vi "target_gas.vi"   [LabVIEW 2011]
uses:
  Input - Cluster gas.ctl
  Output - Cluster gas.ctl
  <vilib>/Platform/TimedLoop/XDataNode/timing_clust.ctl
  <vilib>/Platform/TimedLoop/XDataNode/nitl_modes.ctl
  <vilib>/Platform/TimedLoop/XDataNode/wakeup.ctl
  <vilib>/Platform/TimedLoop/XDataNode/XDataNode.xnode
  <vilib>/Platform/TimedLoop/XDataNode/XDNodeRunTimeDep.lvlib
panel:
  # "The Network Variable Engine and Variable Client Support must be installed on the RT target\nfor this application to function properly. If the Network Variable Engine is not supported on\nthe target (e.g.  FP-2000 with <32MB of RAM), open the project and move the variable library\nto My Computer in the project. Doing this will deploy the variables to localhost but\nwill still require that Variable Client Support be installed on the RT target."
types:
  T1 = cluster{"GA1 ch4 [%]":dbl, "GA1 co2 [%]":dbl, "GA1 h2 [%]":dbl, "empty":bool, "measuring point":u8}
  T2 = typedef "XDNodeRunTimeDep.lvlib/timing_clust.ctl" = cluster{"Expected End [f-1]":u64, "Actual End [f-1]":u64, "Finished Late? [f-1]":bool, "Expected End [i-1]":u64, "Actual End [i-1]":u64, "Finished Late? [i-1]":bool, "Expected Start [i]":u64, "Actual Start [i]":u64, "Expected Start [f]":u64, "Actual Start [f]":u64, "Source Name":string, "Structure Name":string, "Period":i64, "Deadline":i64, "Offset":i64, "Start":i64, "Priority":i32, "Timeout":i32, "Mode":T3, "Wakeup Reason":T4, "Error":errorcluster, "Source Type":string, "Secondary Source Type":string, "Global End Time":u64, "Global Start Time":u64, "Frame Duration":u64, "Iteration Duration":u64, "Assigned CPU":i32, "I/O Scan Engine Mode":u32}
  T3 = typedef "XDNodeRunTimeDep.lvlib/nitl_modes.ctl" = enum32{"No Change", "Process missed periods, maintain original phase", "Discard missed periods, maintain original phase", "Process missed periods, ignore original phase", "Discard missed periods, ignore original phase"}
  T4 = typedef "XDNodeRunTimeDep.lvlib/wakeup.ctl" = enum32{"Normal", "Aborted", "Asynchronous wakeup", "Timing source error", "Timed loop error", "Timeout"}
  T5 = typedef "Input - Cluster gas.ctl" = cluster{"GM P-1":bool, "GM P-2":bool, "measuring point":u32, "measuring mode":u8, "GM-V1,2":bool, "GM-V3,4":bool, "GM-V5":bool, "measuring volume":u32}
  T6 = typedef "Output - Cluster gas.ctl" = cluster{"B2G2 MR V1.1 AUF":bool, "B2G2 MR V1.1 ZU":bool, "B2G2 MR V1 AUF":bool, "B2G2 MR V1 ZU":bool, "B2G1 T2 V1 AUF":bool, "B2G1 T2 V1 ZU":bool, "B2G1 T2 V1.1 AUF":bool, "B2G1 T2 V1.1 ZU":bool, "B2G2 T2 V1 AUF":bool, "B2G2 T2 V1 ZU":bool, "B2G2 T2 V1.1 ZU":bool, "B2G2 T2 V1.1 AUF":bool, "B2G1 MR V1 AUF":bool, "B2G1 MR V1 ZU":bool, "B2G1 MR V1.1 AUF":bool, "B2G1 MR V1.1 ZU":bool, "B2G1 HR V1 AUF":bool, "B2G1 HR V1 ZU":bool, "B2G1 HR V1.1 AUF":bool, "B2G1 HR V1.1 ZU":bool, "Fab1 HR V1 AUF":bool, "Fab1 HR V1 ZU":bool, "Fab1 HR V1.1 AUF":bool, "Fab1 HR V1.1 ZU":bool, "Fab1 MR V1 AUF":bool, "Fab1 MR V1 ZU":bool, "Fab1 MR V1.1 AUF":bool, "Fab1 MR V1.1 ZU":bool, "Fab1 BL V1 AUF":bool, "Fab1 BL V1 ZU":bool, "Fab1 BL V1.1 AUF":bool, "Fab1 BL V1.1 ZU":bool, "Fab2 HR V1 AUF":bool, "Fab2 HR V1 ZU":bool, "Fab2 HR V1.1 AUF":bool, "Fab2 HR V1.1 ZU":bool, "Fab2 MR V1 AUF":bool, "Fab2 MR V1 ZU":bool, "Fab2 MR V1.1 AUF":bool, "Fab2 MR V1.1 ZU":bool, "GA1 ch4 [%]":dbl, "GA1 co2 [%]":dbl, "GA1 h2 [%]":dbl, "GM P1 RUN":bool, "GM V-1 AUF":bool, "GM V-1 ZU":bool, "GM V-2 AUF":bool, "GM V-2 ZU":bool, "GM V-3 AUF":bool, "GM V-3 ZU":bool, "GM V-4 AUF":bool, "GM V-4 ZU":bool, "GM P2 RUN":bool, "GM GZ-1 [imp]":u32, "GM DS-2 [bar]":dbl, "GM DS-1 [bar]":dbl, "GM TS-1 [°C]":dbl, "GM TS-2[°C]":dbl, "gas_values":cluster{"timestamp":timestamp, "GM DS-2 [bar]":dbl, "GA1 ch4 [%]":dbl, "GA1 co2 [%]":dbl, "GA1 h2 [%]":dbl, "GM DS-1 [bar]":dbl, "GM TS-1 [°C]":dbl, "GM TS-2 [°C]":dbl, "GM GZ-1 [l]":dbl, "empty":bool, "measuring point":u8}, "measuring mode":u8}
  T7 = cluster{"STOP":bool, "measuring point":u32, "measuring mode t-1":u8, "measuring mode t-2":u8, "measuring volume":u32, "gas_values":cluster{"GA1 ch4 [%]":dbl, "GA1 co2 [%]":dbl, "GA1 h2 [%]":dbl, "empty":bool, "measuring point":u8}}
  T8 = cluster{"timestamp":timestamp, "GM DS-2 [bar]":dbl, "GA1 ch4 [%]":dbl, "GA1 co2 [%]":dbl, "GA1 h2 [%]":dbl, "GM DS-1 [bar]":dbl, "GM TS-1 [°C]":dbl, "GM TS-2 [°C]":dbl, "GM GZ-1 [l]":dbl, "empty":bool, "measuring point":u8}
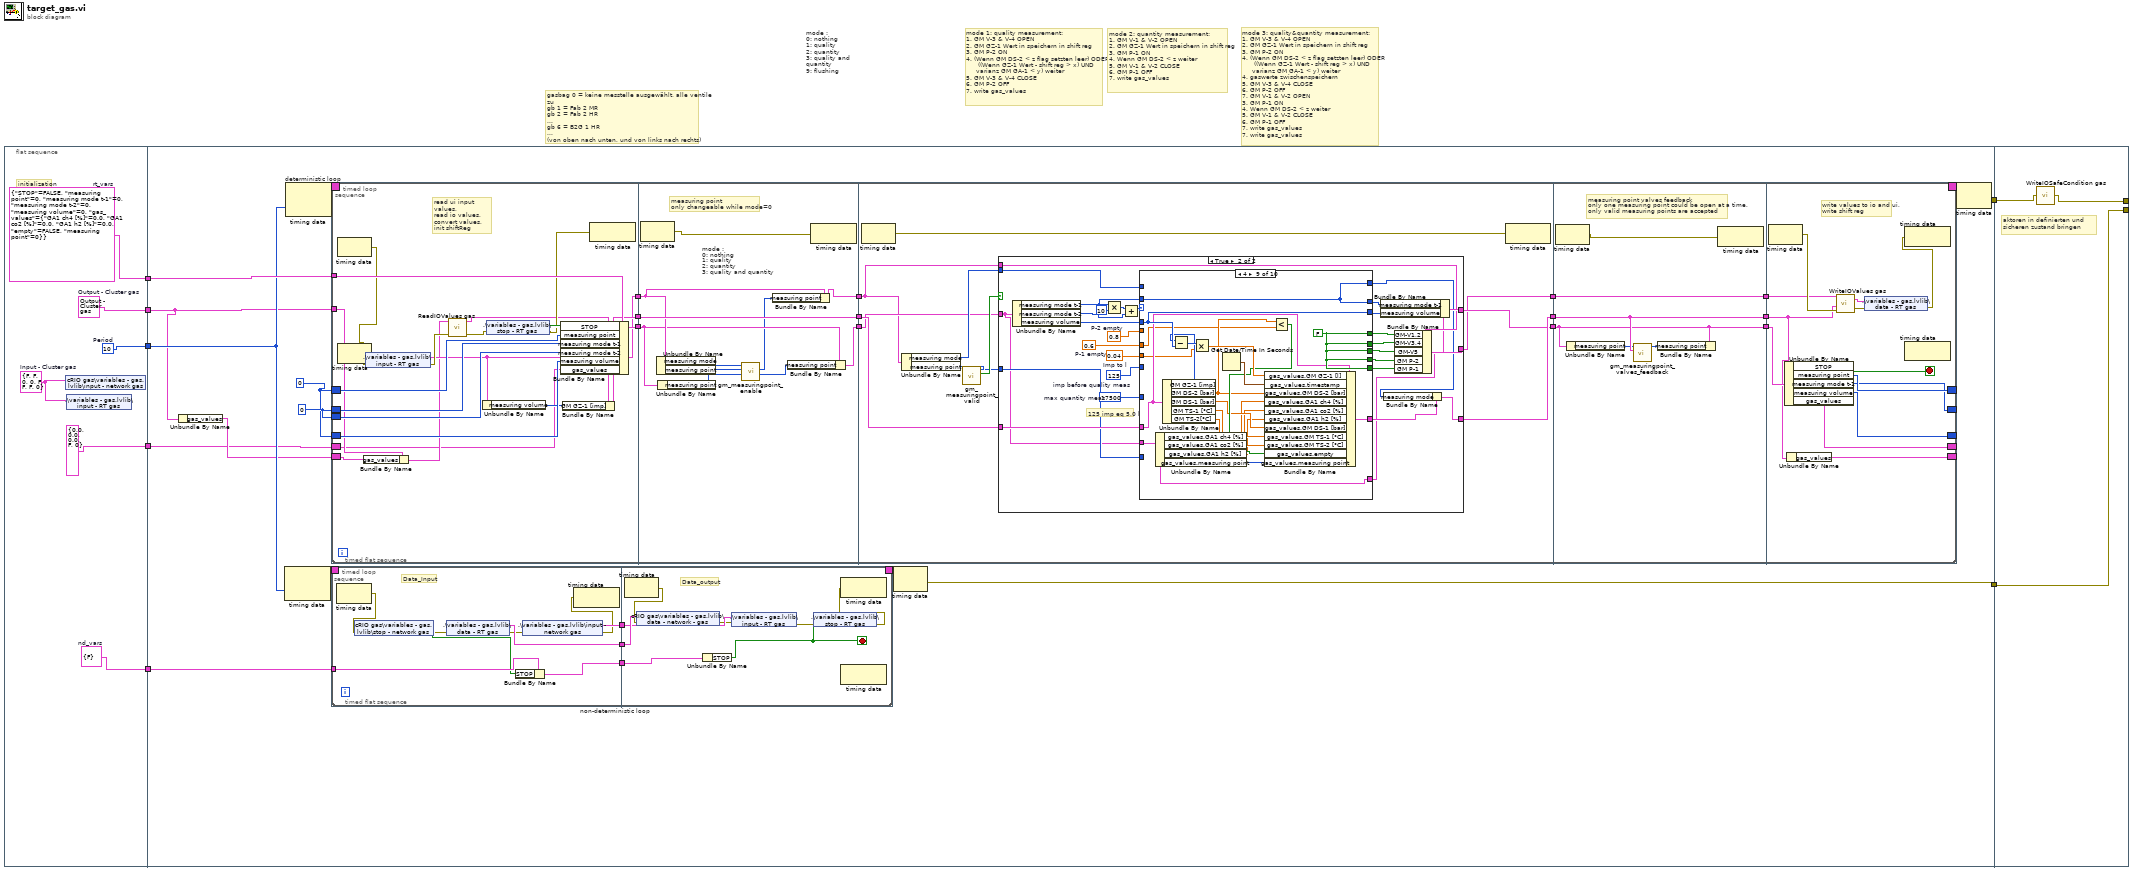
[diagram p0: block diagram]
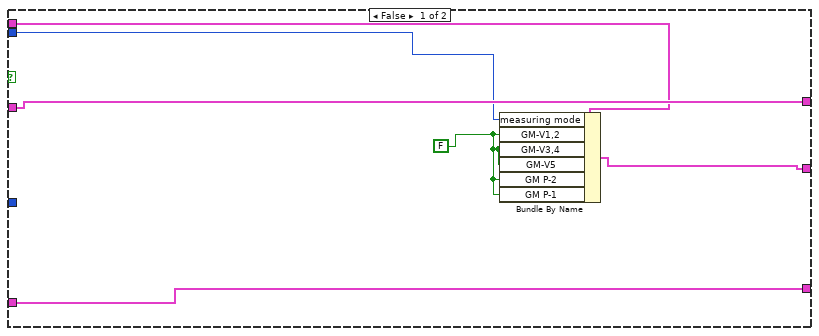
[diagram p2: hidden frame]
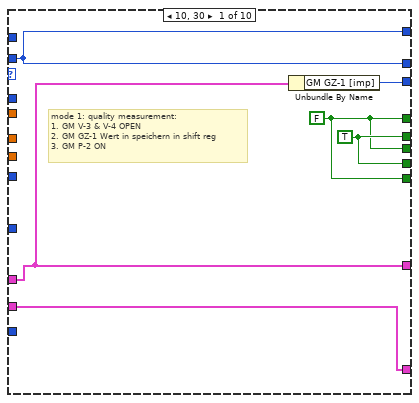
[diagram p3: hidden frame]
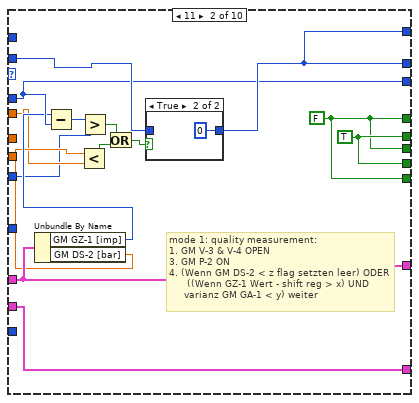
[diagram p4: hidden frame]
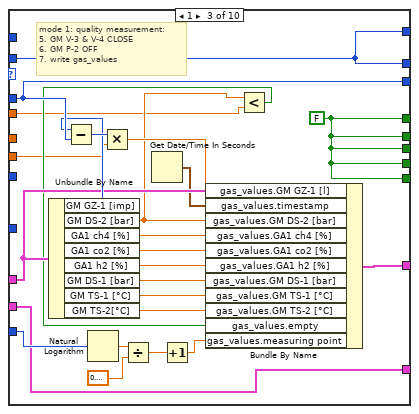
[diagram p6: hidden frame]
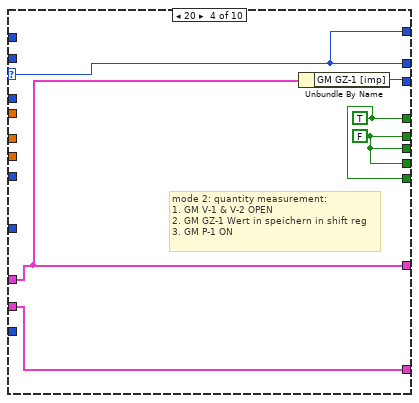
[diagram p7: hidden frame]
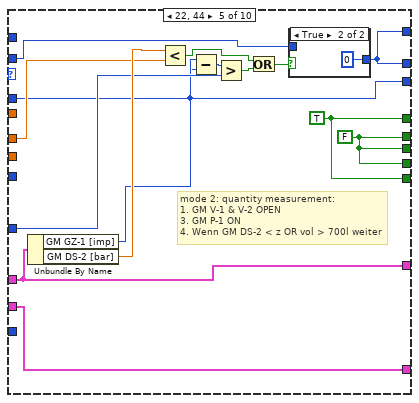
[diagram p8: hidden frame]
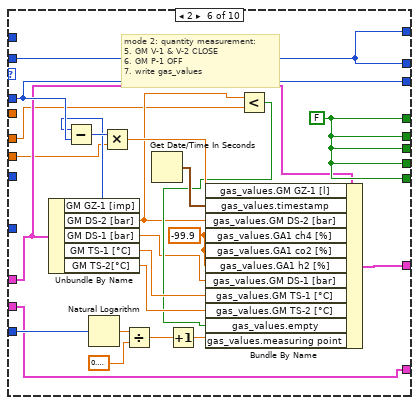
[diagram p10: hidden frame]
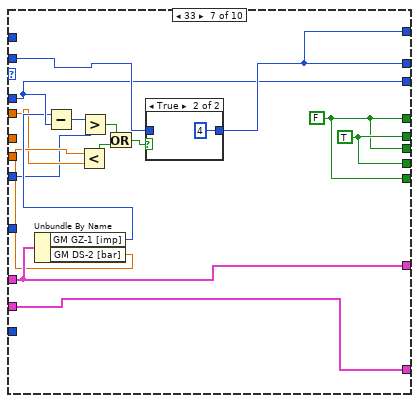
[diagram p11: hidden frame]
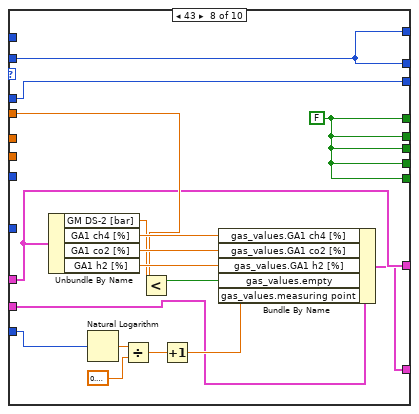
[diagram p13: hidden frame]
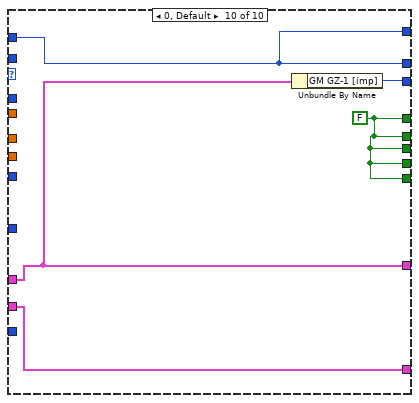
[diagram p14: hidden frame]
diagram:
  # "mode 3: quality&quantity measurement:\n1. GM V-3 & V-4 OPEN\n2. GM GZ-1 Wert in speichern in shift reg\n3. GM P-2 ON\n4. (Wenn GM DS-2 < z flag setzten leer) ODER\n      ((Wenn GZ-1 Wert - shift reg > x) UND\n     varianz GM GA-1 < y) weiter\n4. gaswerte zwischenspeichern\n5. GM V-3 & V-4 CLOSE\n6. GM P-2 OFF\n7. GM V-1 & V-2 OPEN\n3. GM P-1 ON\n4. Wenn GM DS-2 < z weiter\n5. GM V-1 & V-2 CLOSE\n6. GM P-1 OFF\n7. write gas_values\n7. write gas_values"
  # "mode 2: quantity measurement:\n1. GM V-1 & V-2 OPEN\n2. GM GZ-1 Wert in speichern in shift reg\n3. GM P-1 ON\n4. Wenn GM DS-2 < z weiter\n5. GM V-1 & V-2 CLOSE\n6. GM P-1 OFF\n7. write gas_values"
  # "mode :\n0: nothing\n1: quality\n2: quantity\n3: quality and quantity\n9: flushing"
  # "mode 1: quality measurement:\n1. GM V-3 & V-4 OPEN\n2. GM GZ-1 Wert in speichern in shift reg\n3. GM P-2 ON\n4. (Wenn GM DS-2 < z flag setzten leer) ODER\n      ((Wenn GZ-1 Wert - shift reg > x) UND\n     varianz GM GA-1 < y) weiter\n5. GM V-3 & V-4 CLOSE\n6. GM P-2 OFF\n7. write gas_values"
  # "gasbag 0 = keine messtelle ausgewählt, alle ventile zu\ngb 1 = Fab 2 MR\ngb 2 = Fab 2 HR \n...\ngb 6 = B2G 1 HR\n...\n(von oben nach unten, und von links nach rechts)"
  n1 = flat-sequence {
    tunnel: [w13] -> w7
    tunnel: [w12] -> w6
    tunnel: [w11] -> w5
    tunnel: [w9] -> w2
    tunnel: [T1 {"GA1 ch4 [%]"=0.0, "GA1 co2 [%]"=0.0, "GA1 h2 [%]"=0.0, "empty"=FALSE, "measuring point"=0} ("gas_values")] -> w1
    tunnel: w7 -> [w23]
    tunnel: w6 -> [w22]
    tunnel: w5 -> [w16]
    tunnel: [w21] -> w4
    tunnel: [w20] -> w3
    tunnel: w2 -> [w19]
    tunnel: w1 -> [w14]
    tunnel: w4 -> [w388]
    tunnel: w3 -> [w386]
    tunnel: [w387] -> _
    tunnel: [w388] -> _
    frame #0 {
      w9 = cluster{"STOP":bool} {"STOP"=FALSE}  # nd_vars
      w10 = T5 {"GM P-1"=FALSE, "GM P-2"=FALSE, "measuring point"=0, "measuring mode"=0, "GM-V1,2"=FALSE, "GM-V3,4"=FALSE, "GM-V5"=FALSE, "measuring volume"=0}  # Input - Cluster gas
      w11 = T6 {"B2G2 MR V1.1 AUF"=FALSE, "B2G2 MR V1.1 ZU"=FALSE, "B2G2 MR V1 AUF"=FALSE, "B2G2 MR V1 ZU"=FALSE, "B2G1 T2 V1 AUF"=FALSE, "B2G1 T2 V1 ZU"=FALSE, "B2G1 T2 V1.1 AUF"=FALSE, "B2G1 T2 V1.1 ZU"=FALSE, "B2G2 T2 V1 AUF"=FALSE, "B2G2 T2 V1 ZU"=FALSE, "B2G2 T2 V1.1 ZU"=FALSE, "B2G2 T2 V1.1 AUF"=FALSE, "B2G1 MR V1 AUF"=FALSE, "B2G1 MR V1 ZU"=FALSE, "B2G1 MR V1.1 AUF"=FALSE, "B2G1 MR V1.1 ZU"=FALSE, "B2G1 HR V1 AUF"=FALSE, "B2G1 HR V1 ZU"=FALSE, "B2G1 HR V1.1 AUF"=FALSE, "B2G1 HR V1.1 ZU"=FALSE, "Fab1 HR V1 AUF"=FALSE, "Fab1 HR V1 ZU"=FALSE, "Fab1 HR V1.1 AUF"=FALSE, "Fab1 HR V1.1 ZU"=FALSE, "Fab1 MR V1 AUF"=FALSE, "Fab1 MR V1 ZU"=FALSE, "Fab1 MR V1.1 AUF"=FALSE, "Fab1 MR V1.1 ZU"=FALSE, "Fab1 BL V1 AUF"=FALSE, "Fab1 BL V1 ZU"=FALSE, "Fab1 BL V1.1 AUF"=FALSE, "Fab1 BL V1.1 ZU"=FALSE, "Fab2 HR V1 AUF"=FALSE, "Fab2 HR V1 ZU"=FALSE, "Fab2 HR V1.1 AUF"=FALSE, "Fab2 HR V1.1 ZU"=FALSE, "Fab2 MR V1 AUF"=FALSE, "Fab2 MR V1 ZU"=FALSE, "Fab2 MR V1.1 AUF"=FALSE, "Fab2 MR V1.1 ZU"=FALSE, "GA1 ch4 [%]"=0.0, "GA1 co2 [%]"=0.0, "GA1 h2 [%]"=0.0, "GM P1 RUN"=FALSE, "GM V-1 AUF"=FALSE, "GM V-1 ZU"=FALSE, "GM V-2 AUF"=FALSE, "GM V-2 ZU"=FALSE, "GM V-3 AUF"=FALSE, "GM V-3 ZU"=FALSE, "GM V-4 AUF"=FALSE, "GM V-4 ZU"=FALSE, "GM P2 RUN"=FALSE, "GM GZ-1 [imp]"=0, "GM DS-2 [bar]"=0.0, "GM DS-1 [bar]"=0.0, "GM TS-1 [°C]"=0.0, "GM TS-2[°C]"=0.0, "gas_values"={"timestamp"=timestamp(0 s since 1904-01-01), "GM DS-2 [bar]"=0.0, "GA1 ch4 [%]"=0.0, "GA1 co2 [%]"=0.0, "GA1 h2 [%]"=0.0, "GM DS-1 [bar]"=0.0, "GM TS-1 [°C]"=0.0, "GM TS-2 [°C]"=0.0, "GM GZ-1 [l]"=0.0, "empty"=FALSE, "measuring point"=0}, "measuring mode"=0}  # Output - Cluster gas
      w13 = T7 {"STOP"=FALSE, "measuring point"=0, "measuring mode t-1"=0, "measuring mode t-2"=0, "measuring volume"=0, "gas_values"={"GA1 ch4 [%]"=0.0, "GA1 co2 [%]"=0.0, "GA1 h2 [%]"=0.0, "empty"=FALSE, "measuring point"=0}}  # rt_vars
      w12 = i64 10  # Period
      # "initialization"
      n2 = shared-variable "cRIO gas\\variables - gas.lvlib\\input - network gas"(w10) -> ()  [unwired: 1 in, 1 out]
      n3 = shared-variable ".\\variables - gas.lvlib\\input - RT gas"(w10) -> ()  [unwired: 1 in, 1 out]
    }
    frame #1 {
      w18 = u8 0 ("measuring point")
      w17 = u32 0 ("measuring point")
      n4 = Unbundle By Name(w16) -> ("gas_values"=w15:T8)
      n5 = node-c288 ("Input Node")(w22) -> (w25:T2)  [unwired: 1 in]
      n6 = node-c288 ("Input Node")(w22) -> (w27:T2)  [unwired: 1 in]
      n7 = timed-loop "non-deterministic loop" {
        timing: w25 -> [_]
        timing-out: [_] -> w24
        tunnel: w19 -> [w28]
        stop <- w51 stop-if-true
        n8 = timed-sequence {
          timing: _ -> [_]
          timing-out: _ -> [_]
          tunnel: w28 -> [w30]
          n9 = timed-flat-sequence {
            tunnel: [w38] -> w32
            tunnel: [w39] -> w31
            tunnel: w30 -> [w41]
            tunnel: [w40] -> w29
            tunnel: w31 -> [w52]
            tunnel: w32 -> [w53]
            tunnel: w29 -> [w54]
            frame #0 {
              # "Data_Input"
              n10 = node-c288() -> (w36:errorcluster)  [unwired: 1 in]
              n11 = shared-variable "cRIO gas\\variables - gas.lvlib\\stop - network gas"(error in=w36) -> (w37:bool, error out=w35:errorcluster)
              n12 = shared-variable ".\\variables - gas.lvlib\\data - RT gas"(error in=w35) -> (w38:T6, error out=w34:errorcluster)
              n13 = Bundle By Name(cluster=w41, "STOP"=w37) -> (w40:cluster{"STOP":bool})
              n14 = shared-variable ".\\variables - gas.lvlib\\input - network gas"(error in=w34) -> (w39:T5, error out=w33:errorcluster)
              n15 = node-c288(w33) -> ()  [unwired: 1 out]
            }
            frame #1 {
              # "Data_output"
              n16 = node-c288() -> (w50:errorcluster)  [unwired: 1 in]
              n17 = shared-variable "cRIO gas\\variables - gas.lvlib\\data - network - gas"(w53, error in=w50) -> (error out=w49:errorcluster)
              n18 = Unbundle By Name(w54) -> ("STOP"=w51:bool)
              n19 = shared-variable ".\\variables - gas.lvlib\\input - RT gas"(w52, error in=w49) -> (error out=w48:errorcluster)
              n20 = shared-variable ".\\variables - gas.lvlib\\stop - RT gas"(w51, error in=w48) -> (error out=w47:errorcluster)
              n21 = node-c288(w47) -> ()  [unwired: 1 out]
            }
          }
        }
        n22 = node-c288() -> ()  [unwired: 1 in, 1 out]
        n23 = node-c288() -> ()  [unwired: 1 in, 1 out]
      }
      n24 = timed-loop "deterministic loop" {
        timing: w27 -> [_]
        timing-out: [_] -> w26
        tunnel: w23 -> [w79]
        tunnel: w16 -> [w78]
        shift-right: [w77] -> _
        shift-left: w17 -> [w76]
        shift-right: [w75] -> _
        shift-left: w18 -> [w74]
        shift-left: w18 -> [w73]
        shift-right: [w72] -> _
        shift-left: w17 -> [w71]
        shift-right: [w70] -> _
        shift-left: w15 -> [w69]
        shift-right: [w68] -> _
        shift-left: w14 -> [w67]
        stop <- w370 stop-if-true
        n25 = timed-sequence {
          timing: _ -> [_]
          timing-out: _ -> [_]
          tunnel: w79 -> [w104]
          tunnel: w78 -> [w103]
          tunnel: [w96] -> w77
          tunnel: w76 -> [w95]
          tunnel: [w88] -> w75
          tunnel: w74 -> [w87]
          tunnel: w73 -> [w86]
          tunnel: [w85] -> w72
          tunnel: w71 -> [w84]
          tunnel: [w83] -> w70
          tunnel: w69 -> [w82]
          tunnel: [w81] -> w68
          tunnel: w67 -> [w80]
          n26 = timed-flat-sequence {
            tunnel: w104 -> [w123]
            tunnel: w103 -> [w108]
            tunnel: [w110] -> w102
            tunnel: [w119] -> w101
            tunnel: [w111] -> w100
            tunnel: w95 -> [w115]
            tunnel: w87 -> [w114]
            tunnel: w86 -> [w113]
            tunnel: w84 -> [w112]
            tunnel: w82 -> [w106]
            tunnel: w80 -> [w105]
            tunnel: w102 -> [w137]
            tunnel: [w130] -> w94
            tunnel: w101 -> [w134]
            tunnel: [w132] -> w92
            tunnel: w100 -> [w139]
            tunnel: [w139] -> w90
            tunnel: w94 -> [w147]
            tunnel: [w146] -> w93
            tunnel: w92 -> [w149]
            tunnel: [w148] -> w91
            tunnel: w90 -> [w151]
            tunnel: [w150] -> w89
            tunnel: w93 -> [w355]
            tunnel: [w355] -> w99
            tunnel: w91 -> [w350]
            tunnel: [w350] -> w98
            tunnel: w89 -> [w353]
            tunnel: [w353] -> w97
            tunnel: w99 -> [w367]
            tunnel: w98 -> [w371]
            tunnel: w97 -> [w363]
            tunnel: [w366] -> w96
            tunnel: [w365] -> w88
            tunnel: [w364] -> w85
            tunnel: [w362] -> w83
            tunnel: [w361] -> w81
            frame #0 {
              # "read ui input values,\nread io values,\nconvert values,\ninit shiftReg"
              n27 = node-c288 ("Output Node")() -> (w117:errorcluster)  [unwired: 1 in]
              n28 = Bundle By Name(cluster=w108, "gas_values"=w106) -> (w107:T6)
              n29 = shared-variable ".\\variables - gas.lvlib\\input - RT gas"(error in=w117) -> (w110:T5, error out=w116:errorcluster)
              n30 = call "ReadIOValues gas.vi"("error in"=w116, "Output - Cluster gas"=w107) -> ("error out"=w120:errorcluster, "Output - Cluster gas"=w118:T6)  [unwired: 2 in]
              n31 = Unbundle By Name(w110) -> ("measuring volume"=w109:u32)
              n32 = shared-variable ".\\variables - gas.lvlib\\stop - RT gas"(error in=w120) -> (w122:bool, error out=w121:errorcluster)
              n33 = Bundle By Name(cluster=w123, "STOP"=w122, "measuring point"=w115, "measuring mode t-1"=w114, "measuring mode t-2"=w113, "measuring volume"=w112, "gas_values"=w105) -> (w119:T7)
              n34 = Bundle By Name(cluster=w118, "GM GZ-1 [imp]"=w109) -> (w111:T6)
              n35 = node-c288 ("Input Node")(w121) -> ()  [unwired: 1 out]
            }
            frame #1 {
              # "mode :\n0: nothing\n1: quality\n2: quantity\n3: quality and quantity"
              # "measuring point\nonly changeable while mode=0"
              n36 = node-c288() -> (w138:errorcluster)  [unwired: 1 in]
              n37 = Unbundle By Name(w137) -> ("measuring mode"=w136:u8, "measuring point"=w135:u32)
              n38 = Unbundle By Name(w134) -> ("measuring point"=w133:u32)
              n39 = call "gm_measuringpoint_enable.vi"("shift reg"=w133, "measuring point"=w135, "measuring mode"=w136) -> ("shift reg out"=w131:u32, "measuring point"=w129:u32)  [unwired: 6 in]
              n40 = Bundle By Name(cluster=w137, "measuring point"=w129) -> (w130:T5)
              n41 = Bundle By Name(cluster=w134, "measuring point"=w131) -> (w132:T7)
              n42 = node-c288(w138) -> ()  [unwired: 1 out]
            }
            frame #2 {
              n43 = node-c288() -> (w155:errorcluster)  [unwired: 1 in]
              n44 = Unbundle By Name(w147) -> ("measuring mode"=w152:u8, "measuring point"=w153:u32)
              n45 = call "gm_measuringpoint_valid.vi"("measuring point in"=w153) -> ("Boolean"=w154:bool, "measuring point out"=w145:u32)  [unwired: 9 in]
              n46 = case shown="True" w154 {
                tunnel: w152 -> [w156 w190]
                tunnel: w151 -> [w161 w186]
                tunnel: [w161 w171] -> w150
                tunnel: w149 -> [w160 w163]
                tunnel: [w160 w182] -> w148
                tunnel: w147 -> [w159 w174]
                tunnel: [w158 w173] -> w146
                tunnel: w145 -> [_ w169]
                frame False {
                  w157 = FALSE ("GM-V3,4")
                  n47 = Bundle By Name(cluster=w159, "measuring mode"=w156, "GM-V1,2"=w157, "GM-V3,4"=w157, "GM-V5"=w157, "GM P-2"=w157, "GM P-1"=w157) -> (w158:T5)
                }
                frame True {
                  w164 = u32 17500  # max quantity meas
                  w165 = u32 125  # imp before quality meas
                  w166 = 0.6  # P-1 empty
                  w167 = 0.8  # P-2 empty
                  w168 = 0.04  # Imp to l
                  # "125 imp eq 5,0 l"
                  n48 = Unbundle By Name(w163) -> ("measuring mode t-1"=w185:u8, "measuring mode t-2"=w184:u8, "measuring volume"=w183:u32)
                  n49 = Multiply(x=w185, y=u8 10) -> (x*y=w189:u8)
                  n50 = Add(x=w189, y=w184) -> (x+y=w188:u8)
                  n51 = case shown="4" w188 {
                    selector: w188 -> [_ _ _ w244 _ _ _ _ _ _]
                    tunnel: w190 -> [_ _ _ _ _ _ _ _ _ w344]
                    tunnel: [w194 w208 w237 w244 w257 w283 w296 w317 w338 w344] -> w181
                    tunnel: [w195 w210 w238 w243 w259 w284 w298 w318 w339 w343] -> w179
                    tunnel: [w196 w211 w238 w242 w254 w284 w299 w318 w339 w343] -> w178
                    tunnel: [w195 w210 w238 w242 w254 w284 w298 w318 w339 w343] -> w177
                    tunnel: [w194 w208 w237 w244 w257 w283 w296 w317 w338 w344] -> w170
                    tunnel: [w192 w207 w236 w240 w247 w282 w295 w316 w337 w341] -> w180
                    tunnel: [w196 w211 w238 w242 w254 w284 w299 w318 w339 w343] -> w176
                    tunnel: [w195 w210 w238 w243 w259 w284 w298 w318 w339 w343] -> w175
                    tunnel: w183 -> [_ w207 w236 _ w247 w282 w295 w316 w337 _]
                    tunnel: w185 -> [w194 w209 w237 _ w258 w283 w297 w317 w338 _]
                    tunnel: w186 -> [w193 w202 w232 w241 w256 w278 w290 w304 w333 w342]
                    tunnel: [w193 w202 w233 w241 w256 w279 w290 w304 w334 w342] -> w172
                    tunnel: w169 -> [_ _ w221 _ _ w267 _ w309 _ _]
                    tunnel: w168 -> [_ _ w216 _ _ w263 _ _ w324 _]
                    tunnel: w167 -> [_ w199 w215 _ _ _ w287 w305 _ _]
                    tunnel: w166 -> [_ _ _ _ w253 w264 _ _ w325 _]
                    tunnel: w165 -> [_ w198 _ _ _ _ w286 _ _ _]
                    tunnel: w164 -> [_ _ _ _ w249 _ _ _ _ _]
                    tunnel: w163 -> [w191 w197 w214 w239 w245 w262 w285 w303 w323 w340]
                    tunnel: [w191 w197 w214 w239 w245 w262 w285 w302 w323 w340] -> w162
                    frame 10, 30 {
                      w195 = FALSE ("GM-V3,4")
                      w196 = TRUE ("GM-V3,4")
                      # "mode 1: quality measurement:\n1. GM V-3 & V-4 OPEN\n2. GM GZ-1 Wert in speichern in shift reg\n3. GM P-2 ON"
                      n52 = Unbundle By Name(w193) -> ("GM GZ-1 [imp]"=w192:u32)
                    }
                    frame 11 {
                      w210 = FALSE ("GM-V3,4")
                      w211 = TRUE ("GM-V3,4")
                      # "mode 1: quality measurement:\n1. GM V-3 & V-4 OPEN\n3. GM P-2 ON\n4. (Wenn GM DS-2 < z flag setzten leer) ODER\n      ((Wenn GZ-1 Wert - shift reg > x) UND\n     varianz GM GA-1 < y) weiter"
                      n53 = Unbundle By Name(w202) -> ("GM GZ-1 [imp]"=w201:u32, "GM DS-2 [bar]"=w200:dbl)
                      n54 = Subtract(x=w201, y=w207) -> (x-y=w206:u32)
                      n55 = Less?(x=w200, y=w199) -> (x < y?=w203:bool)
                      n56 = Greater?(x=w206, y=w198) -> (0:w204:bool)
                      n57 = Or(x=w204, y=w203) -> (x .or. y?=w205:bool)
                      n58 = case shown="True" w205 {
                        tunnel: w209 -> [w212 _]
                        tunnel: [w212 u8 0 ("measuring mode t-1")] -> w208
                        frame False {
                        }
                        frame True {
                        }
                      }
                    }
                    frame 1 {
                      w238 = FALSE ("GM-V3,4")
                      # "mode 1: quality measurement:\n5. GM V-3 & V-4 CLOSE\n6. GM P-2 OFF\n7. write gas_values"
                      n59 = Unbundle By Name(w232) -> ("GM GZ-1 [imp]"=w234:u32, "GM DS-2 [bar]"=w218:dbl, "GA1 ch4 [%]"=w229:dbl, "GA1 co2 [%]"=w228:dbl, "GA1 h2 [%]"=w227:dbl, "GM DS-1 [bar]"=w217:dbl, "GM TS-1 [°C]"=w226:dbl, "GM TS-2[°C]"=w225:dbl)
                      n60 = Subtract(x=w234, y=w236) -> (x-y=w235:u32)
                      n61 = Natural Logarithm(1:w221) -> (0:w223:dbl)
                      n62 = Multiply(x=w235, y=w216) -> (x*y=w230:dbl)
                      n63 = Divide(x=w223, y=0.6931471805599453) -> (x/y=w220:dbl)
                      n64 = Get Date/Time In Seconds ("timestamp")() -> (seconds since 1Jan1904=w231:timestamp)
                      n65 = Increment(x=w220) -> (x+1=w219:dbl)
                      n66 = Less?(x=w218, y=w215) -> (x < y?=w224:bool)
                      n67 = Bundle By Name(cluster=w232, "gas_values.GM GZ-1 [l]"=w230, "gas_values.timestamp"=w231, "gas_values.GM DS-2 [bar]"=w218, "gas_values.GA1 ch4 [%]"=w229, "gas_values.GA1 co2 [%]"=w228, "gas_values.GA1 h2 [%]"=w227, "gas_values.GM DS-1 [bar]"=w217, "gas_values.GM TS-1 [°C]"=w226, "gas_values.GM TS-2 [°C]"=w225, "gas_values.empty"=w224, "gas_values.measuring point"=w219) -> (w233:T6)
                    }
                    frame 20 {
                      w242 = FALSE ("GM-V3,4")
                      w243 = TRUE ("GM-V3,4")
                      # "mode 2: quantity measurement:\n1. GM V-1 & V-2 OPEN\n2. GM GZ-1 Wert in speichern in shift reg\n3. GM P-1 ON"
                      n68 = Unbundle By Name(w241) -> ("GM GZ-1 [imp]"=w240:u32)
                    }
                    frame 22, 44 {
                      w259 = TRUE ("GM-V3,4")
                      w254 = FALSE ("GM-V3,4")
                      # "mode 2: quantity measurement:\n1. GM V-1 & V-2 OPEN\n3. GM P-1 ON\n4. Wenn GM DS-2 < z OR vol > 700l weiter"
                      n69 = Unbundle By Name(w256) -> ("GM GZ-1 [imp]"=w248:u32, "GM DS-2 [bar]"=w255:dbl)
                      n70 = Less?(x=w255, y=w253) -> (x < y?=w252:bool)
                      n71 = Subtract(x=w248, y=w247) -> (x-y=w250:u32)
                      n72 = Greater?(x=w250, y=w249) -> (0:w246:bool)
                      n73 = Or(x=w252, y=w246) -> (x .or. y?=w251:bool)
                      n74 = case shown="True" w251 {
                        tunnel: w258 -> [w260 _]
                        tunnel: [w260 u8 0 ("measuring mode t-1")] -> w257
                        frame False {
                        }
                        frame True {
                        }
                      }
                    }
                    frame 2 {
                      w272 = -99.9 ("gas_values.GA1 ch4 [%]")
                      w284 = FALSE ("GM-V3,4")
                      # "mode 2: quantity measurement:\n5. GM V-1 & V-2 CLOSE\n6. GM P-1 OFF\n7. write gas_values"
                      n75 = Unbundle By Name(w278) -> ("GM GZ-1 [imp]"=w280:u32, "GM DS-2 [bar]"=w266:dbl, "GM DS-1 [bar]"=w265:dbl, "GM TS-1 [°C]"=w275:dbl, "GM TS-2[°C]"=w274:dbl)
                      n76 = Subtract(x=w280, y=w282) -> (x-y=w281:u32)
                      n77 = Natural Logarithm(1:w267) -> (0:w271:dbl)
                      n78 = Multiply(x=w281, y=w263) -> (x*y=w276:dbl)
                      n79 = Divide(x=w271, y=0.6931471805599453) -> (x/y=w269:dbl)
                      n80 = Get Date/Time In Seconds ("timestamp")() -> (seconds since 1Jan1904=w277:timestamp)
                      n81 = Increment(x=w269) -> (x+1=w268:dbl)
                      n82 = Less?(x=w266, y=w264) -> (x < y?=w273:bool)
                      n83 = Bundle By Name(cluster=w278, "gas_values.GM GZ-1 [l]"=w276, "gas_values.timestamp"=w277, "gas_values.GM DS-2 [bar]"=w266, "gas_values.GA1 ch4 [%]"=w272, "gas_values.GA1 co2 [%]"=w272, "gas_values.GA1 h2 [%]"=w272, "gas_values.GM DS-1 [bar]"=w265, "gas_values.GM TS-1 [°C]"=w275, "gas_values.GM TS-2 [°C]"=w274, "gas_values.empty"=w273, "gas_values.measuring point"=w268) -> (w279:T6)
                    }
                    frame 33 {
                      w298 = FALSE ("GM-V3,4")
                      w299 = TRUE ("GM-V3,4")
                      n84 = Unbundle By Name(w290) -> ("GM GZ-1 [imp]"=w289:u32, "GM DS-2 [bar]"=w288:dbl)
                      n85 = Subtract(x=w289, y=w295) -> (x-y=w294:u32)
                      n86 = Less?(x=w288, y=w287) -> (x < y?=w291:bool)
                      n87 = Greater?(x=w294, y=w286) -> (0:w292:bool)
                      n88 = Or(x=w292, y=w291) -> (x .or. y?=w293:bool)
                      n89 = case shown="True" w293 {
                        tunnel: w297 -> [w300 _]
                        tunnel: [w300 u8 4 ("measuring mode t-1")] -> w296
                        frame False {
                        }
                        frame True {
                        }
                      }
                    }
                    frame 43 {
                      w318 = FALSE ("GM-V3,4")
                      n90 = Unbundle By Name(w304) -> ("GM DS-2 [bar]"=w306:dbl, "GA1 ch4 [%]"=w315:dbl, "GA1 co2 [%]"=w314:dbl, "GA1 h2 [%]"=w313:dbl)
                      n91 = Natural Logarithm(1:w309) -> (0:w311:dbl)
                      n92 = Divide(x=w311, y=0.6931471805599453) -> (x/y=w308:dbl)
                      n93 = Less?(x=w306, y=w305) -> (x < y?=w312:bool)
                      n94 = Increment(x=w308) -> (x+1=w307:dbl)
                      n95 = Bundle By Name(cluster=w303, "gas_values.GA1 ch4 [%]"=w315, "gas_values.GA1 co2 [%]"=w314, "gas_values.GA1 h2 [%]"=w313, "gas_values.empty"=w312, "gas_values.measuring point"=w307) -> (w302:T7)
                    }
                    frame 4 {
                      w339 = FALSE ("GM-V3,4")
                      n96 = Unbundle By Name(w323) -> ("gas_values.GA1 ch4 [%]"=w321:dbl, "gas_values.GA1 co2 [%]"=w320:dbl, "gas_values.GA1 h2 [%]"=w319:dbl, "gas_values.measuring point"=w322:u8)
                      n97 = Unbundle By Name(w333) -> ("GM GZ-1 [imp]"=w335:u32, "GM DS-2 [bar]"=w327:dbl, "GM DS-1 [bar]"=w326:dbl, "GM TS-1 [°C]"=w330:dbl, "GM TS-2[°C]"=w329:dbl)
                      n98 = Subtract(x=w335, y=w337) -> (x-y=w336:u32)
                      n99 = Multiply(x=w336, y=w324) -> (x*y=w331:dbl)
                      n100 = Get Date/Time In Seconds ("timestamp")() -> (seconds since 1Jan1904=w332:timestamp)
                      n101 = Less?(x=w327, y=w325) -> (x < y?=w328:bool)
                      n102 = Bundle By Name(cluster=w333, "gas_values.GM GZ-1 [l]"=w331, "gas_values.timestamp"=w332, "gas_values.GM DS-2 [bar]"=w327, "gas_values.GA1 ch4 [%]"=w321, "gas_values.GA1 co2 [%]"=w320, "gas_values.GA1 h2 [%]"=w319, "gas_values.GM DS-1 [bar]"=w326, "gas_values.GM TS-1 [°C]"=w330, "gas_values.GM TS-2 [°C]"=w329, "gas_values.empty"=w328, "gas_values.measuring point"=w322) -> (w334:T6)
                    }
                    frame 0, Default {
                      w343 = FALSE ("GM-V3,4")
                      n103 = Unbundle By Name(w342) -> ("GM GZ-1 [imp]"=w341:u32)
                    }
                  }
                  n104 = Bundle By Name(cluster=w162, "measuring mode t-1"=w181, "measuring volume"=w180) -> (w182:T7)
                  n105 = Bundle By Name(cluster=w172, "measuring mode"=w170) -> (w171:T6)
                  n106 = Bundle By Name(cluster=w174, "GM-V1,2"=w179, "GM-V3,4"=w178, "GM-V5"=w177, "GM P-2"=w176, "GM P-1"=w175) -> (w173:T5)
                }
              }
              n107 = node-c288(w155) -> ()  [unwired: 1 out]
            }
            frame #3 {
              # "measuring point valves feedback \nonly one measuring point could be open at a time,\nonly valid measuring points are accepted"
              n108 = node-c288() -> (w354:errorcluster)  [unwired: 1 in]
              n109 = Unbundle By Name(w350) -> ("measuring point"=w352:u32)
              n110 = call "gm_measuringpoint_valves_feedback.vi"("Output - Cluster gas"=w353, "measuring point"=w352) -> ("measuring point"=w351:u32)  [unwired: 9 in]
              n111 = Bundle By Name(cluster=w350, "measuring point"=w351) -> ()  [unwired: 1 out]
              n112 = node-c288(w354) -> ()  [unwired: 1 out]
            }
            frame #4 {
              # "write values to io and ui,\nwrite shift reg"
              n113 = node-c288() -> (w369:errorcluster)  [unwired: 1 in]
              n114 = Unbundle By Name(w371) -> ("STOP"=w370:bool, "measuring point"=w366:u32, "measuring mode t-1"=w365:u8, "measuring volume"=w364:u32, "gas_values"=w361:T1)
              n115 = Unbundle By Name(w363) -> ("gas_values"=w362:T8)
              n116 = call "WriteIOValues gas.vi"("error in"=w369, "Output - Cluster gas"=w363, "input cluster"=w367) -> ("error out"=w368:errorcluster, "Output - Cluster gas 2"=w373:T6)  [unwired: 1 in]
              n117 = shared-variable ".\\variables - gas.lvlib\\data - RT gas"(w373, error in=w368) -> (error out=w372:errorcluster)
              n118 = node-c288(w372) -> ()  [unwired: 1 out]
            }
          }
        }
        n119 = node-c288() -> ()  [unwired: 1 in, 1 out]
        n120 = node-c288() -> ()  [unwired: 1 in, 1 out]
      }
      n121 = node-c288 ("Output Node")(w24) -> (w21:errorcluster)
      n122 = node-c288 ("Output Node")(w26) -> (w20:errorcluster)
    }
    frame #2 {
      # "aktoren in definierten und sicheren zustand bringen"
      n123 = call "WriteIOSafeCondition gas.vi"("error in"=w386) -> ("error out"=w387:errorcluster)
    }
  }
